vi "OpenCLV Examples.vi"   [LabVIEW 2012]
uses:
  <vilib>/Platform/browser.llb/Open URL in Default Browser (path).vi
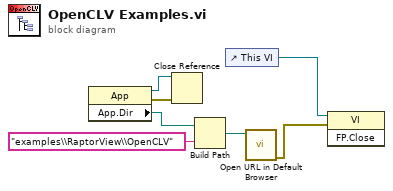
[diagram p0: block diagram]
diagram:
  n1 = property class="App"() -> (reference out=w3:refnum<vi>, error out=w4:errorcluster, "App.Dir"=w5:path)  [unwired: 2 in]
  n2 = Close Reference(reference=w3, error in (no error)=w4) -> ()  [unwired: 1 out]
  n3 = Build Path(base path=w5, name or relative path="examples\\RaptorView\\OpenCLV") -> (appended path=w6:path)
  n4 = control-ref of="This VI"() -> (w2:refnum<vi>)
  n5 = call-poly <vilib>:"Open URL in Default Browser.vi"("path"=w6) -> ("error out"=w1:errorcluster)  [unwired: 5 in, 1 out]
  n6 = invoke class="VI" method="FP.Close"(reference=w2, error in=w1) -> ()  [unwired: 1 in, 3 out]
